vi "Read_coeff.vi"(10 "sos gain SF controller file path":path, 11 "sos coeff file path":path) -> (0 "b02(2)":fxp<+/-,64,9>[](array[numeric]), 1 "b01(2)":fxp<+/-,64,9>[](array[numeric]), 2 "-a02(2)":fxp<+/-,64,9>[](array[numeric]), 3 "-a01(2)":fxp<+/-,64,9>[](array[numeric]), 5 "sos gain SF Controller":fxp<+/-,42,9>)   [LabVIEW 2015]
uses:
  <vilib>/Utility/file.llb/Read Delimited Spreadsheet (DBL).vi
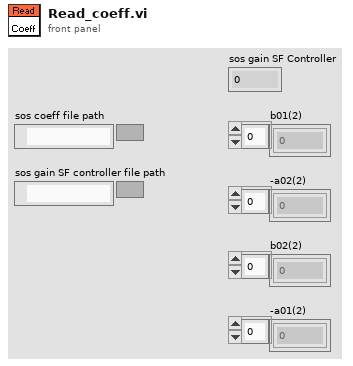
[diagram p1: front panel]
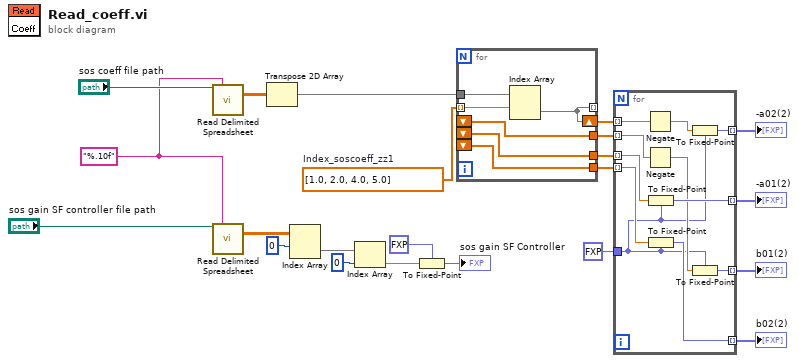
[diagram p0: block diagram]
diagram:
  w1 = "%.10f" ("format (%.3f)")
  w2 = dbl[] [1.0, 2.0, 4.0, 5.0]  # Index_soscoeff_zz1
  n1 = call-poly <vilib>:"Read Delimited Spreadsheet.vi"("file path (dialog if empty)"="sos coeff file path", "format (%.3f)"=w1) -> ("all rows"=w13:dbl[][])  [unwired: 8 in, 5 out]
  n2 = call-poly <vilib>:"Read Delimited Spreadsheet.vi"("file path (dialog if empty)"="sos gain SF controller file path", "format (%.3f)"=w1) -> ("all rows"=w20:dbl[][])  [unwired: 8 in, 5 out]
  n3 = Transpose 2D Array(2D array=w13) -> (transposed array=w3:dbl[][])
  n4 = Index Array(array=w20, index (row)=0 ("index (row) 10")) -> (element=w14:dbl[])  [unwired: 1 in]
  n5 = Index Array(array=w14, index=0 ("index (row) 11")) -> (element=w16:dbl)
  n6 = To Fixed-Point(fixed-point type=fxp<+/-,42,9> 0.0 ("fixed-point type 2"), number=w16) -> (fixed-point=→"sos gain SF Controller":fxp<+/-,42,9>)
  n7 = for {
    tunnel: w2 -> [w28] mode=indexing
    tunnel: w3 -> [w27]
    tunnel: [w26] -> _ mode=indexing
    shift-right: [w26] -> w11
    shift-left: _ -> [w25]
    shift-left: _ -> [w24]
    shift-left: _ -> [w23]
    tunnel: [w25] -> w10
    tunnel: [w24] -> w9
    tunnel: [w23] -> w8
    n8 = Index Array "Index Array"(array=w27, index (row)=w28) -> (element=w26:dbl[])  [unwired: 1 in]
  }
  n9 = for {
    tunnel: w10 -> [w39] mode=indexing
    tunnel: [w38] -> w4 mode=indexing
    tunnel: w11 -> [w37] mode=indexing
    tunnel: w8 -> [w36] mode=indexing
    tunnel: w9 -> [w35] mode=indexing
    tunnel: [w34] -> w5 mode=indexing
    tunnel: [w33] -> w6 mode=indexing
    tunnel: [w32] -> w7 mode=indexing
    tunnel: fxp<+/-,64,9> 0.0 ("fixed-point type") -> [w29]
    n10 = Negate(x=w37) -> (-x=w30:dbl)
    n11 = Negate(x=w39) -> (-x=w31:dbl)
    n12 = To Fixed-Point(fixed-point type=w29, number=w35) -> (fixed-point=w32:fxp<+/-,64,9>)
    n13 = To Fixed-Point(fixed-point type=w29, number=w36) -> (fixed-point=w33:fxp<+/-,64,9>)
    n14 = To Fixed-Point(fixed-point type=w29, number=w30) -> (fixed-point=w34:fxp<+/-,64,9>)
    n15 = To Fixed-Point(fixed-point type=w29, number=w31) -> (fixed-point=w38:fxp<+/-,64,9>)
  }
  "-a01(2)" <- w7
  "b02(2)" <- w6
  "-a02(2)" <- w5
  "b01(2)" <- w4
